vi "Program list Selection.vi"(8 "error in":errorcluster, 10 "Filepath":path=path "D:/My Project/2019-2020/Magnetic Mareli UM/MM_UM/Project Setup/data/program seq/Program_280A.bin", 11 "vi referenceIn":refnum<vi>) -> (0 "error out":errorcluster, 1 "Exit":bool, 2 "String":string, 3 "vi reference Out":refnum<vi>)   [LabVIEW 2020]
uses:
  Control Button/Exit.ctl
  Control Button/next.ctl
  Galobal variable_TI.vi
  <vilib>/addons/database/Connection.llb/DB Tools Open Connec (String).vi
  <vilib>/addons/database/_DB Variant To Data/Database Variant To Data.xnode
  <vilib>/addons/database/NI_Database_API.lvlib
panel:
  in  "Cluster 3":T1
  out "error out 3":errorcluster
  out "error out 2":errorcluster
  out "String 2":string
  in  "Next":T2
  in  "Exit":T3
  in  "Program List":string(combo)
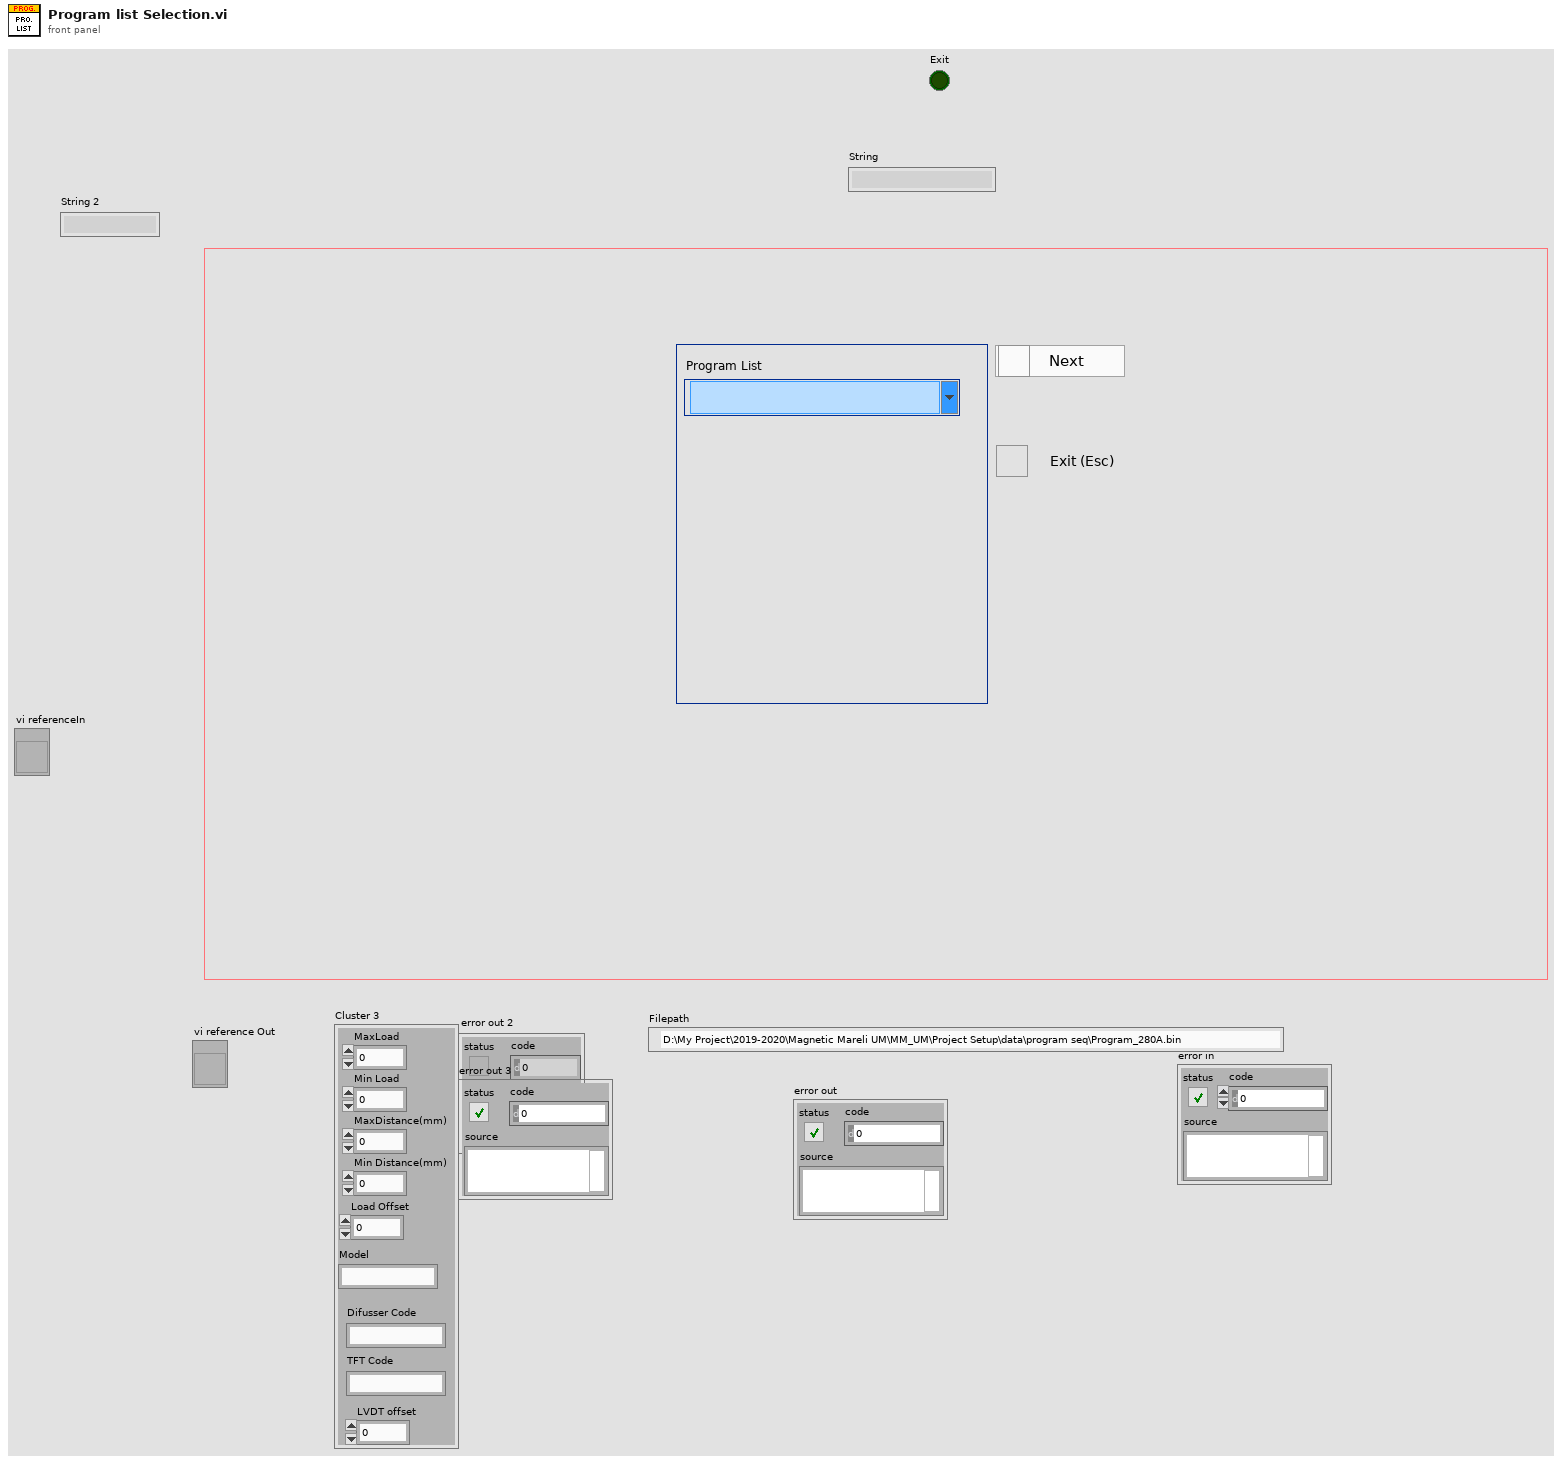
[diagram p1: front panel]
types:
  T1 = cluster{"MaxLoad ":dbl, "Min Load":dbl, "MaxDistance(mm)":dbl, "Min Distance(mm)":dbl, "Load Offset":dbl, "Model":string, "Difusser Code":string, "TFT Code ":string, "LVDT offset":dbl}
  T2 = typedef "next.ctl" = bool
  T3 = typedef "Exit.ctl" = bool
  T4 = enum32{"Invalid", "Standard", "Closed", "Hidden", "Minimized", "Maximized"}
  T5 = typedef "NI_Database_API.lvlib/Conn ObjectReference.ctl" = refnum<k1>
  T6 = cluster{"MaxLoad ":dbl, "Min Load":dbl, "MaxDistance(mm)":dbl, "Min Distance(mm)":dbl, "Load Offset":dbl, "Model":string, "Difusser Code":string, "TFT Code ":string, "Load Offset 2":dbl}
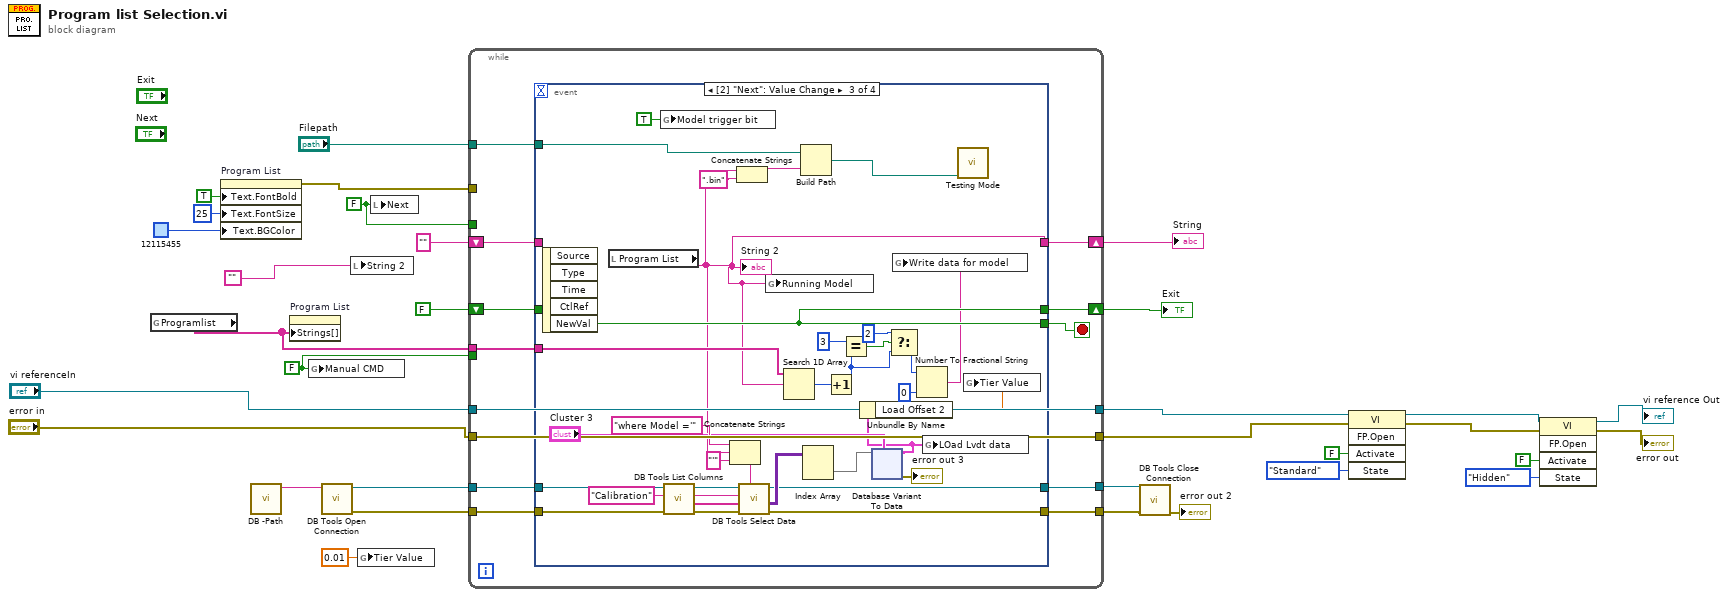
[diagram p0: block diagram]
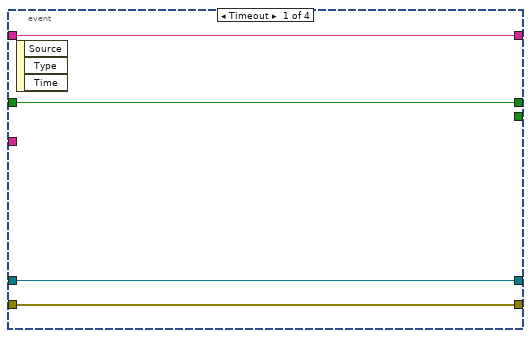
[diagram p2: hidden frame]
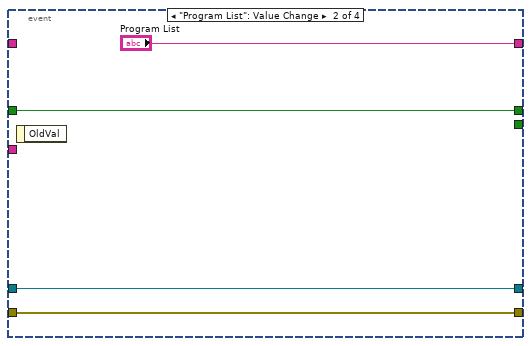
[diagram p3: hidden frame]
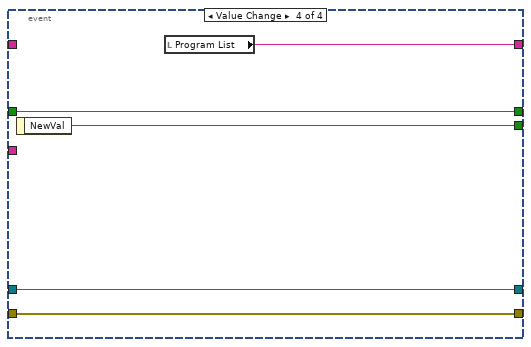
[diagram p4: hidden frame]
diagram:
  w21 = FALSE ("Manual CMD")
  w22 = FALSE ("Next")
  n1 = global read "Galobal variable_TI.vi" "Programlist"() -> (w28:string[])
  n2 = property on="Program List" class="CmbBox"("Text.FontBold"=TRUE ("Text.Font:Bold"), "Text.FontSize"=u32 25 ("Text.Font:Size"), "Text.BGColor"=u32 12115455 ("Color Box")) -> (error out=w25:errorcluster)  [unwired: 2 in, 1 out]
  n3 = call "DB -Path.vi"() -> ("String"=w19:string)  [unwired: 11 in]
  n4 = property on="Program List" class="CmbBox"("Strings[]"=w28) -> ()  [unwired: 2 in, 2 out]
  n5 = global write "Galobal variable_TI.vi" "Manual CMD"(w21) -> ()
  n6 = call-poly <vilib>:"DB Tools Open Connection.vi"("connection information"=w19) -> ("error out"=w17:errorcluster, "connection reference"=w18:T5)  [unwired: 7 in]
  n7 = local write "String 2"("") -> ()
  n8 = global write "Galobal variable_TI.vi" "Tier Value"(0.01 ("Tier Value")) -> ()
  n9 = local write "Next"(w22) -> ()
  n10 = while {
    shift-right: [w45] -> w32
    shift-left: "" ("Combo Box") -> [w44]
    shift-right: [w42] -> w29
    shift-left: T3 FALSE ("NewVal") -> [w41]
    tunnel: w28 -> [w33]
    tunnel: w25 -> [_]
    tunnel: w22 -> [_]
    tunnel: w21 -> [_]
    tunnel: "vi referenceIn" -> [w40]
    tunnel: [w40] -> w5
    tunnel: "error in" -> [w39]
    tunnel: [w39] -> w4
    tunnel: "Filepath" -> [w38]
    tunnel: w18 -> [w37]
    tunnel: w17 -> [w36]
    tunnel: [w35] -> w16
    tunnel: [w34] -> w15
    stop <- w43 stop-if-true
    n11 = event shown="[2] \"Next\": Value Change" {
      selector: _ -> [_ _ _ _]
      dyn-events: _ -> [_ _ _ _]
      timeout: _ -> [_ _ _ _]
      tunnel: [w49 "Program List" w65 w373] -> w45
      tunnel: w44 -> [w49 _ _ _]
      tunnel: [_ _ w86 w374] -> w43
      tunnel: [w48 w52 w86 w372] -> w42
      tunnel: w41 -> [w48 w52 _ w372]
      tunnel: w38 -> [_ _ w83 _]
      tunnel: w37 -> [w47 w51 w72 w371]
      tunnel: w36 -> [w46 w50 w71 w370]
      tunnel: [w47 w51 w70 w371] -> w35
      tunnel: [w46 w50 w69 w370] -> w34
      tunnel: w33 -> [_ _ w66 _]
      event Timeout {
        n12 = event-data() -> ()  [unwired: 1 in, 3 out]
      }
      event "Program List": Value Change {
        n13 = event-data() -> ()  [unwired: 1 in, 1 out]
      }
      event Value Change {
        w78 = "Calibration" ("table")
        n14 = event-data() -> ("NewVal"=w86:T2)  [unwired: 1 in, 4 out]
        n15 = local read "Program List"() -> (w65:string)
        "String 2" <- w65
        n16 = global write "Galobal variable_TI.vi" "Model trigger bit"(TRUE ("Model trigger bit")) -> ()
        n17 = call <vilib>:"DB Tools List Columns.vi"("error in (no error)"=w71, "table"=w78, "connection reference"=w72) -> ("error out"=w75:errorcluster, "columns"=w77:string[], "connection reference out"=w76:T5)  [unwired: 1 in, 1 out]
        n18 = Concatenate Strings("where Model ='" ("string"), w65, "'" ("string")) -> (w74:string)
        n19 = Concatenate Strings(w65, ".bin" ("string")) -> (w84:string)
        n20 = call <vilib>:"DB Tools Select Data.vi"("condition"=w74, "error in (no error)"=w75, "columns"=w77, "table"=w78, "connection reference"=w76) -> ("error out"=w69:errorcluster, "data"=w73:variant[][], "connection reference out"=w70:T5)  [unwired: 1 in]
        n21 = global write "Galobal variable_TI.vi" "Running Model"(w65) -> ()
        n22 = Search 1D Array(1D array=w66, element=w65) -> (index of element=w64:i32)  [unwired: 1 in]
        n23 = Build Path(base path=w83, name or relative path=w84) -> (appended path=w82:path)
        n24 = Index Array(array=w73) -> (element=w81:variant[])  [unwired: 2 in]
        n25 = Increment(x=w64) -> (x+1=w55:i32)
        n26 = Equal?(x=3, y=w55) -> (x = y?=w57:bool)
        n27 = xnode "Database Variant To Data"("database variant"=w81, "type"="Cluster 3") -> ("data"=w60:T6, "error out"=→"error out 3":errorcluster)  [unwired: 1 in]
        n28 = Unbundle By Name(w60) -> ("Load Offset 2"=w59:dbl)
        n29 = Select(t=2 ("x"), s=w57, f=w55) -> (s? t:f=w54:i32)
        n30 = Number To Fractional String(number=w54, precision (6)=i16 0) -> (F-format string=w63:string)  [unwired: 2 in]
        n31 = global write "Galobal variable_TI.vi" "Write data for model"(w63) -> ()
        n32 = global write "Galobal variable_TI.vi" "LOad Lvdt data"(w60) -> ()
        n33 = call "Testing Mode.vi"("Filepath"=w82) -> ()  [unwired: 10 in, 1 out]
        n34 = global write "Galobal variable_TI.vi" "Tier Value"(w59) -> ()
      }
      event Value Change {
        n35 = event-data() -> ("NewVal"=w374:T3)  [unwired: 1 in]
        n36 = local read "Program List"() -> (w373:string)
      }
    }
  }
  "String" <- w32
  "Exit" <- w29
  n37 = call <vilib>:"DB Tools Close Connection.vi"("error in (no error)"=w15, "connection reference"=w16) -> ("error out"=→"error out 2":errorcluster)  [unwired: 5 in]
  n38 = invoke class="VI" method="FP.Open"(reference=w5, error in=w4, "Activate"=FALSE ("Activate?"), "State"=T4."Standard") -> (reference out=w7:refnum<vi>, error out=w6:errorcluster)  [unwired: 1 in, 3 out]
  n39 = invoke class="VI" method="FP.Open"(reference=w7, error in=w6, "Activate"=FALSE ("Activate?"), "State"=T4."Hidden") -> (reference out=→"vi reference Out":refnum<vi>, error out=→"error out":errorcluster)  [unwired: 1 in, 3 out]
